vi "Assert No Error.vi"(8 "Error":errorcluster) -> (2 "Success":bool)   [LabVIEW 2024]
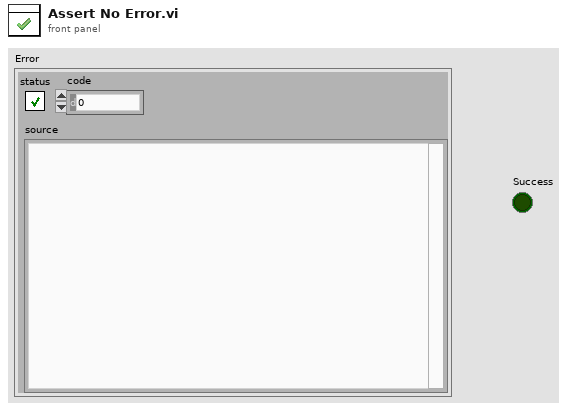
[diagram p1: front panel]
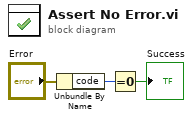
[diagram p0: block diagram]
diagram:
  n1 = Unbundle By Name("Error") -> ("code"=w3:i32)
  n2 = Equal To 0?(x=w3) -> (x = 0?=→"Success":bool)
